vi "KM Lockin.vi"() -> ()   [LabVIEW 2015]
uses:
  MQM Data Transfer_KM.vi
  String Array Select.vi
  <vilib>/Utility/file.llb/Write To Spreadsheet File (string).vi
  Numeric Array Select.vi
  <vilib>/Utility/file.llb/Write To Spreadsheet File (DBL).vi
panel:
  in  "Tab Control":enum32{"Display Data", "Sweep Arming"}(tab)
  in  "Control":bool=TRUE
  in  "Stop":bool=TRUE
  out "XY Graph":cluster{dbl[], dbl[]}[](graph)
  in  "Display Elements":cluster{"X":bool, "Y":bool, "Name":u16}[](array[cluster]) {"Name" items=["Time (ms)", "Field (T)", "Temperature (K)", "", "HFLI_1.0 Freq (Hz)", "HFLI_1.0 R (V)", "HFLI_1.0 Theta (deg)", "HFLI_1.0 X (mV)", "HFLI_1.0 Y (mV)"]}
  in  "X-Axis":u16(ring) items=["Linear", "Reciprocal", "Log10"]
  in  "Filename":path=path "C:/Users/putkonen.CPFS/Dropbox.lvm"
  in  "Delay (ms)":dbl=2000.0
  out "Data Rate (ms)":u32
  in  "Finish":bool
  out "Measurement":bool
  in  "Y-Axis":u16(ring) items=["Linear", "Reciprocal", "Log10"]
  out "Saving":bool
  in  "Data Recording":bool=TRUE
  in  "DAQ time (ms)":u32=500
  out "Circles":cluster{dbl[], dbl[]}(graph)
  in  "X":u16(ring) items=["Linear", "Reciprocal", "Log10"]
  in  "Y":u16(ring) items=["Linear", "Reciprocal", "Log10"]
  out "Phase":cluster{dbl[], dbl[]}(graph)
  in  "Frequency":u16(ring) items=["Linear", "Reciprocal", "Log10"]
  in  "Theta":u16(ring) items=["Linear", "Reciprocal", "Log10"]
  out "# pts in freq sweep":i32
  out "Data Rate  (ms)":u32
  in  "DAQ time (ms)":u32=50
  in  "Fequency sweep datafile":path=path "C:/Users/putkonen.CPFS/Dropbox.lvm" caption="Filename"
  in  "Save current freq scan":bool
  in  "Start (Hz)":dbl=48.29
  in  "Stop (Hz)":dbl=48.57
  in  "# pts in scan":dbl=100.0
  in  "Bandwidth (Hz)":dbl=10.0
  in  "Use Sweep Control":bool
  in  "Sweep Parameter":u16(ring) items=["Temperature", "Field", "Position", "Measure when stable"]
  out "Global Stop":bool
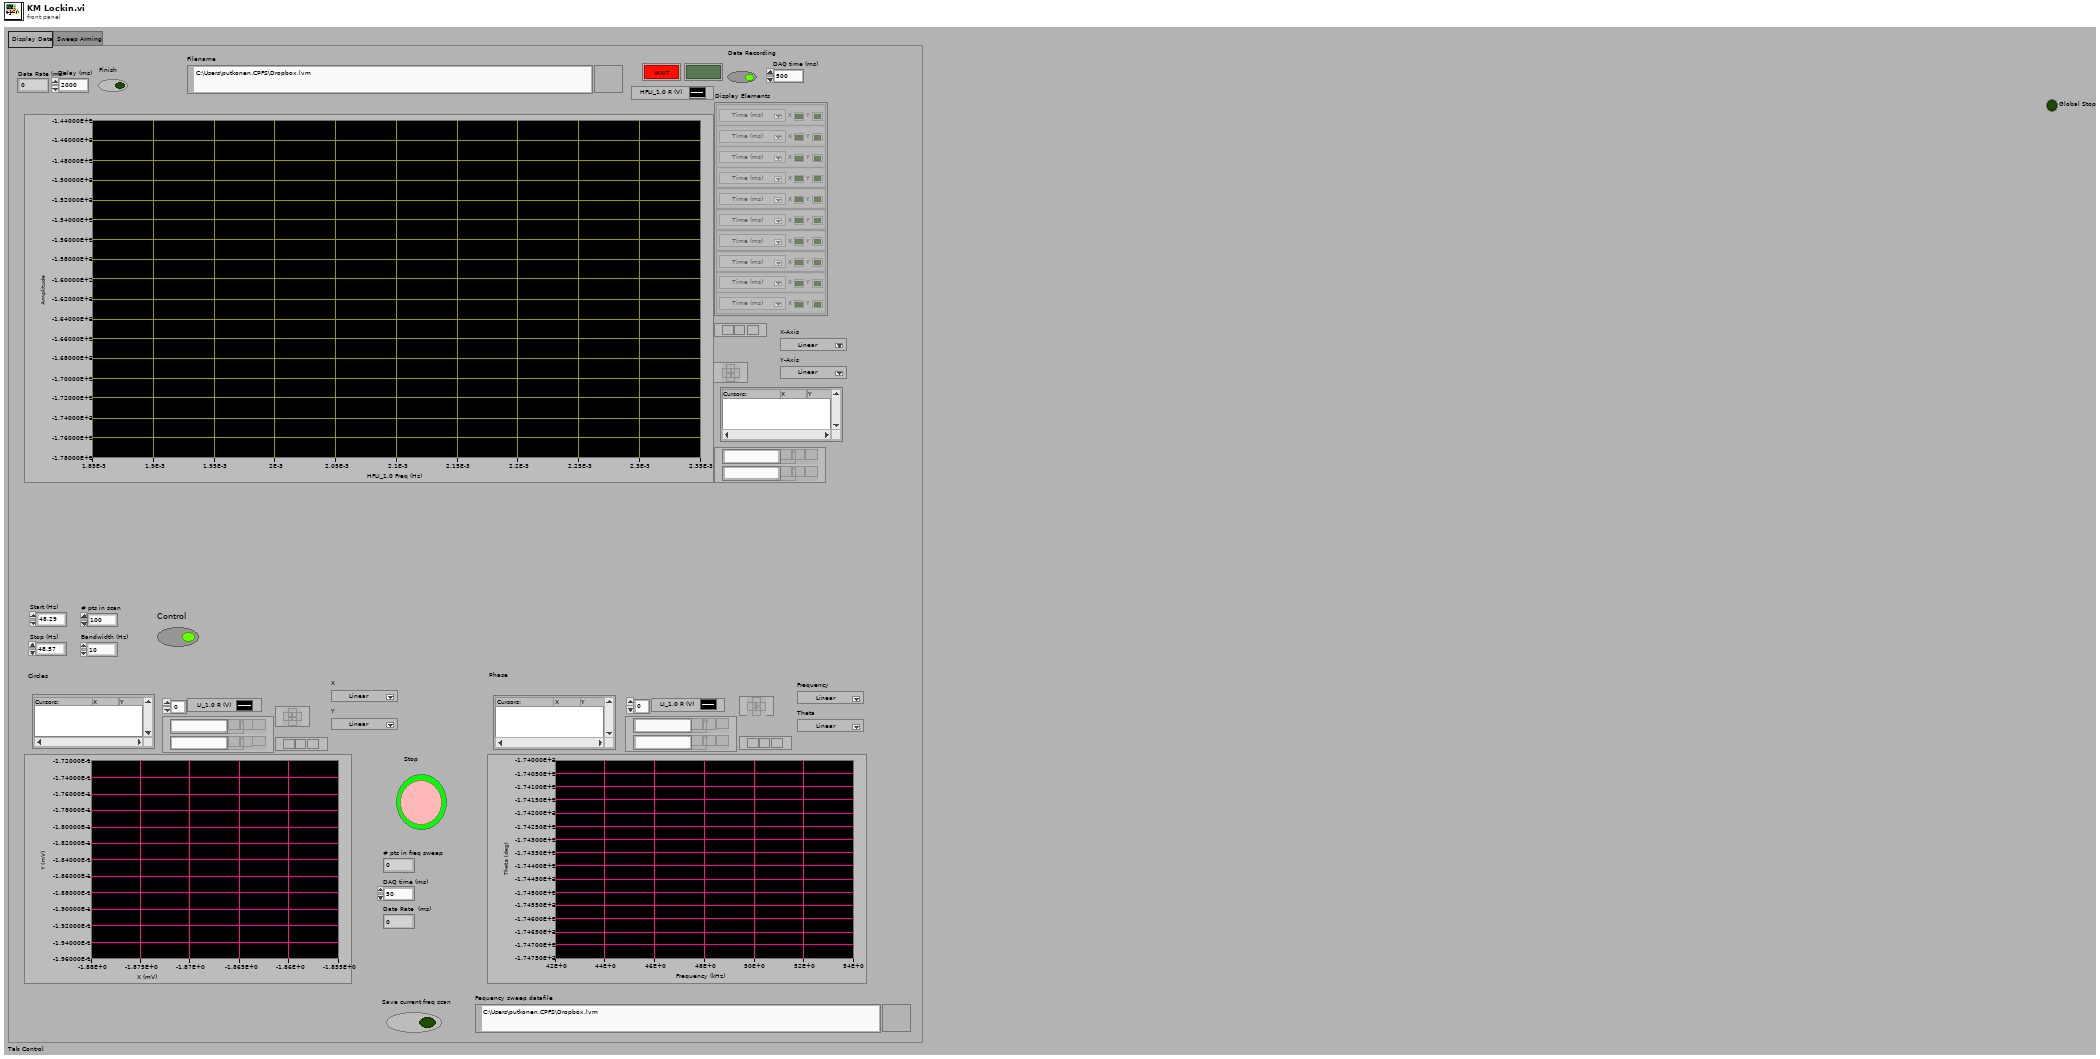
[diagram p1: front panel]
types:
  T1 = typedef "ZI_Frontpanel.ctl" = cluster{"Lockin 1 Demod 0":cluster{"R(V)":dbl, "Theta (deg)":dbl, "Timestamp (ms)":u32}, "Lockin 2 Demod 0":cluster{"R(V)":dbl, "Theta (deg)":dbl, "Timestamp (ms)":u32}, "Lockin 3 Demod 0":cluster{"R(V)":dbl, "Theta (deg)":dbl, "Timestamp (ms)":u32}, "Lockin 4 Demod 0":cluster{"R(V)":dbl, "Theta (deg)":dbl, "Timestamp (ms)":u32}, "Lockin 1 Demod 1":cluster{"R(V)":dbl, "Theta (deg)":dbl, "Timestamp (ms)":u32}, "Lockin 2 Demod 1":cluster{"R(V)":dbl, "Theta (deg)":dbl, "Timestamp (ms)":u32}, "Lockin 3 Demod 1":cluster{"R(V)":dbl, "Theta (deg)":dbl, "Timestamp (ms)":u32}, "Lockin 4 Demod 1":cluster{"R(V)":dbl, "Theta (deg)":dbl, "Timestamp (ms)":u32}, "Lockin 1 Demod 2":cluster{"R(V)":dbl, "Theta (deg)":dbl, "Timestamp (ms)":u32}, "Lockin 1 Demod 3":cluster{"R(V)":dbl, "Theta (deg)":dbl, "Timestamp (ms)":u32}, "LI1 active":bool, "LI2 active":bool, "LI3 active":bool, "LI4 active":bool}
  T2 = typedef "PPMS_Status.ctl" = cluster{"Field":cluster{"Field (T)":dbl, "Field stable":bool, "Timestamp (ms)":u32}, "Temperature":cluster{"Temperature (K)":dbl, "Temperature stable":bool, "Timestamp (ms)":u32}}
  T3 = typedef "Rotator_Status.ctl" = cluster{"Angle (deg)":dbl, "Stopped":bool, "Timestamp (ms)":u32}
  T4 = cluster{"Request new file":bool, "Sweep variable":u16, "Pause DAQ":bool}
  T5 = typedef "HF_FrontPanel.ctl" = cluster{"Lockin 1 Demod 0":cluster{"R(V)":dbl, "Theta (deg)":dbl, "Frequency (Hz)":dbl, "X (mV)":dbl, "Y (mV)":dbl}, "LI1 active":bool, "Timestamp (ms)":u32}
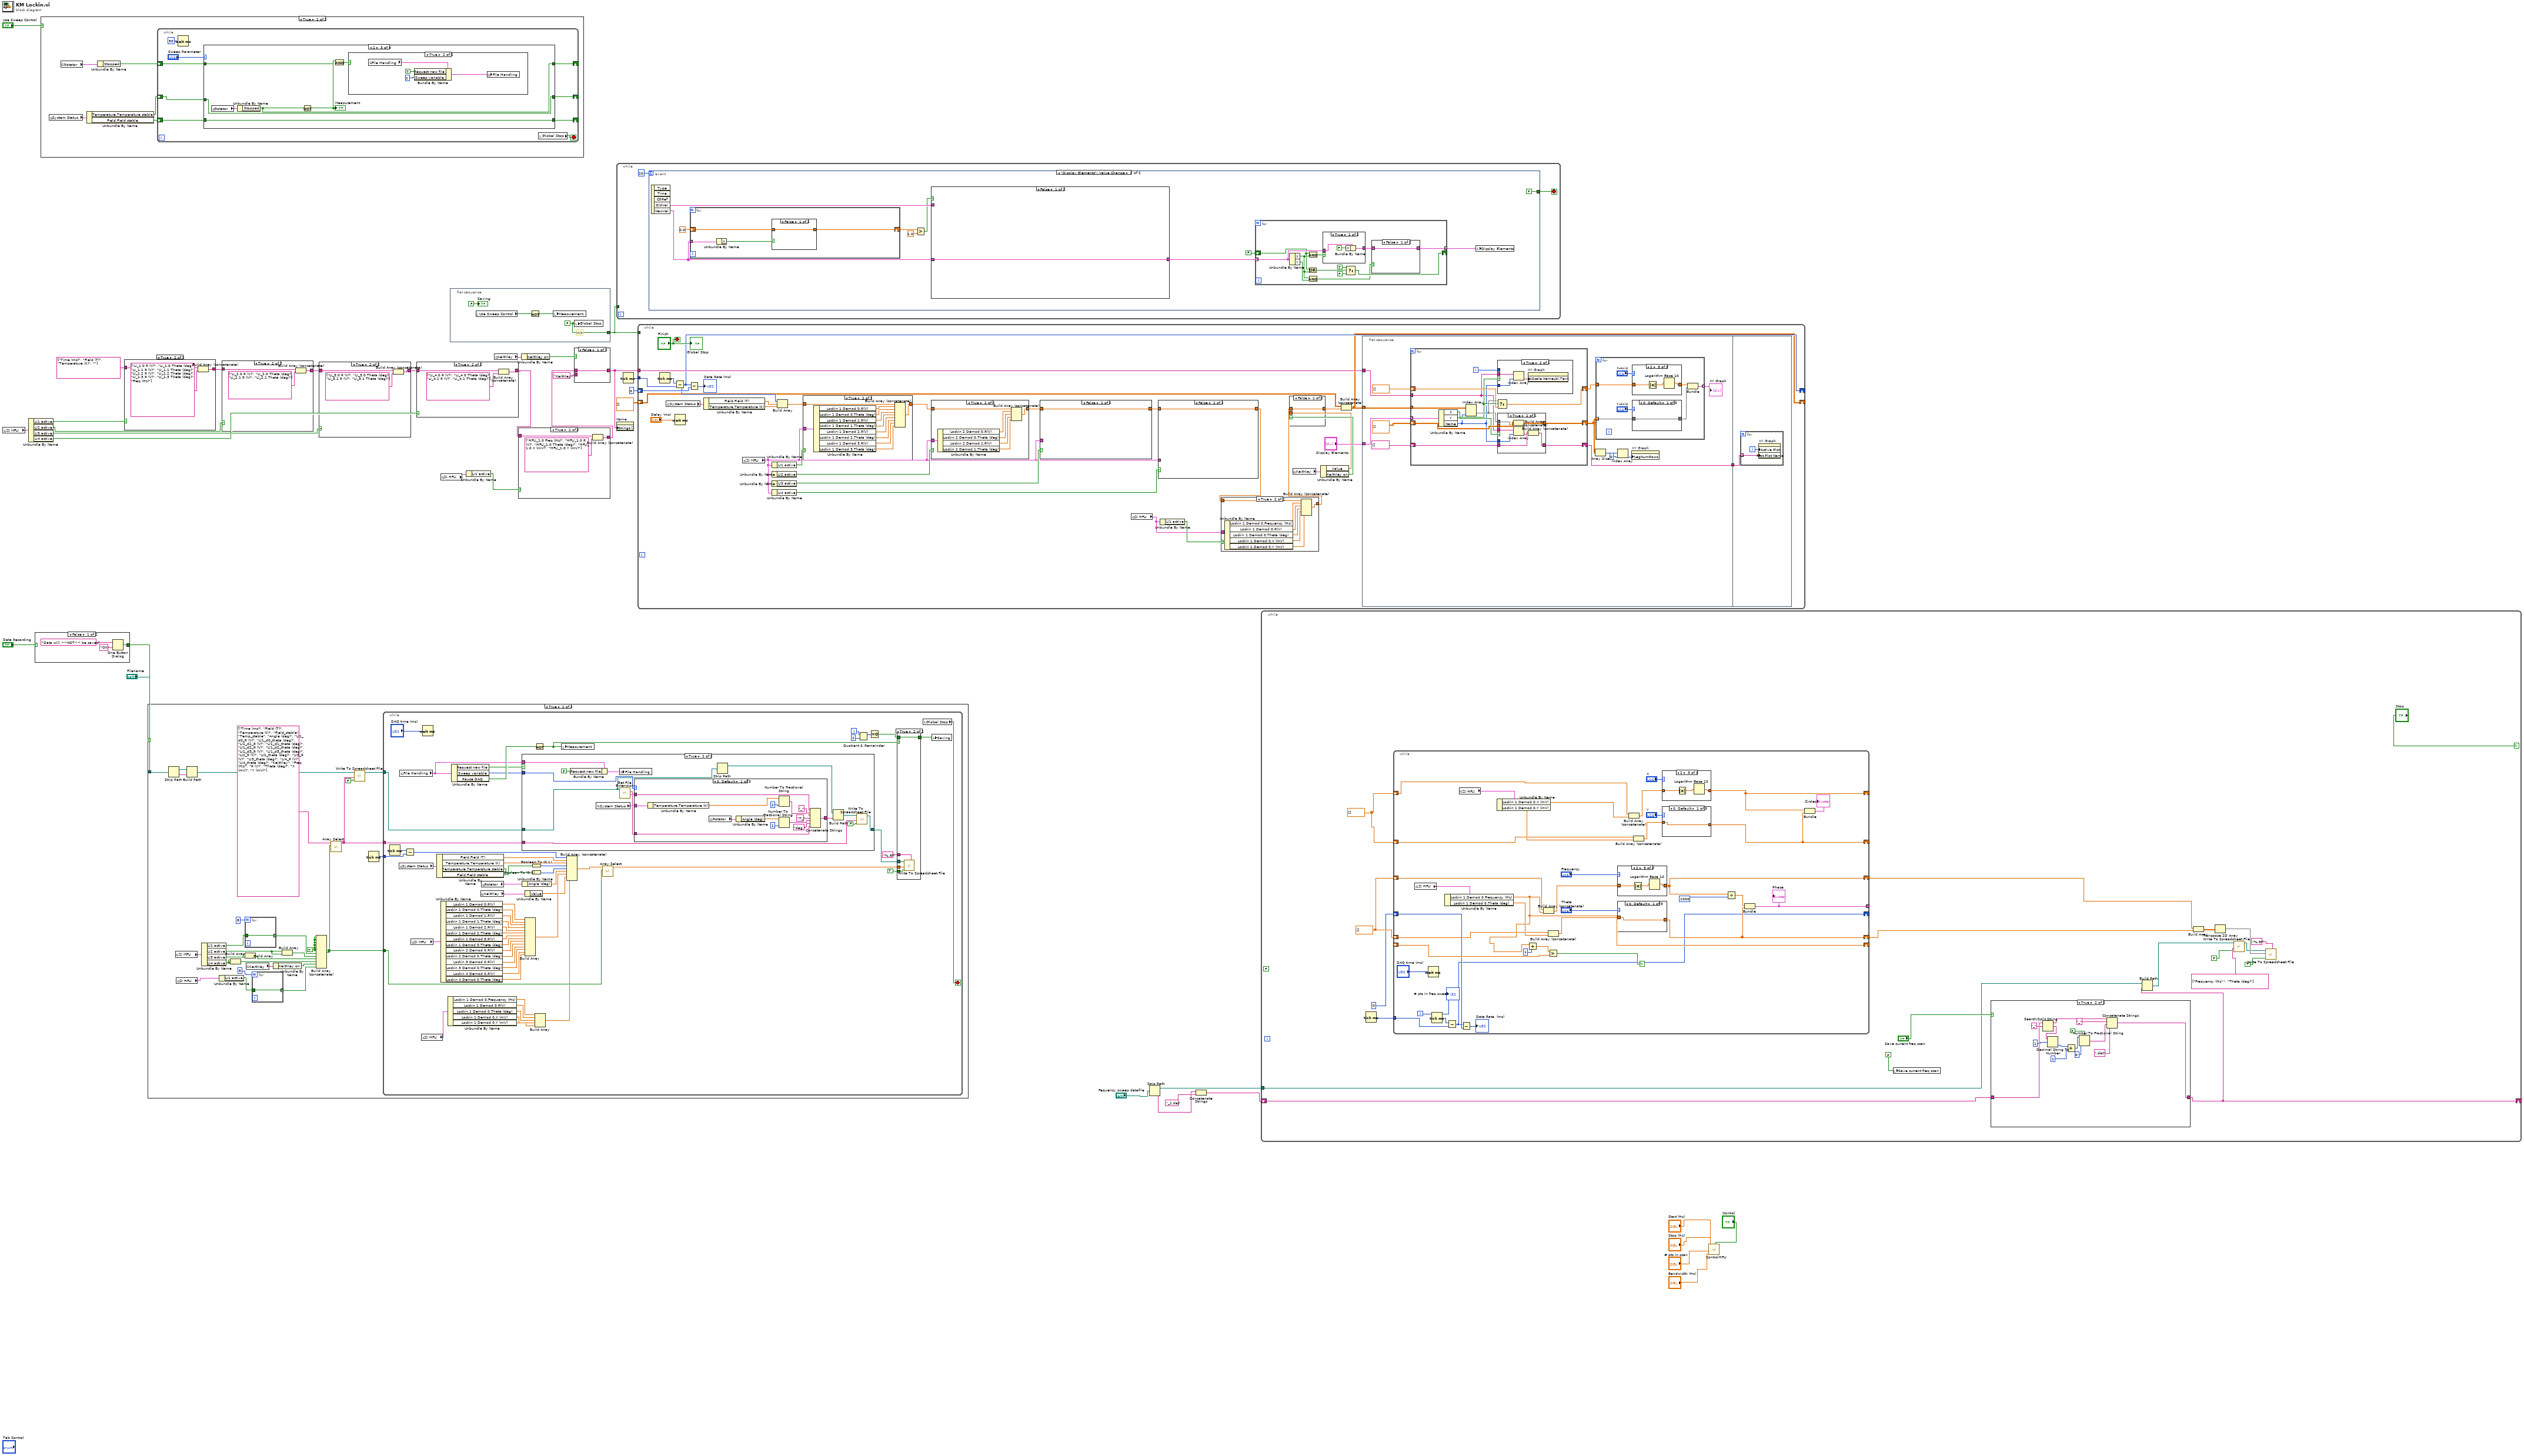
[diagram p0: block diagram]
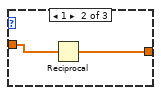
[diagram p3: hidden frame]
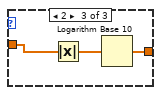
[diagram p4: hidden frame]
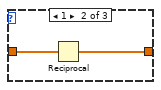
[diagram p6: hidden frame]
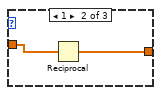
[diagram p7: hidden frame]
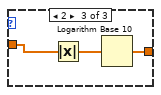
[diagram p8: hidden frame]
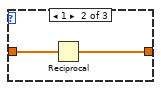
[diagram p10: hidden frame]
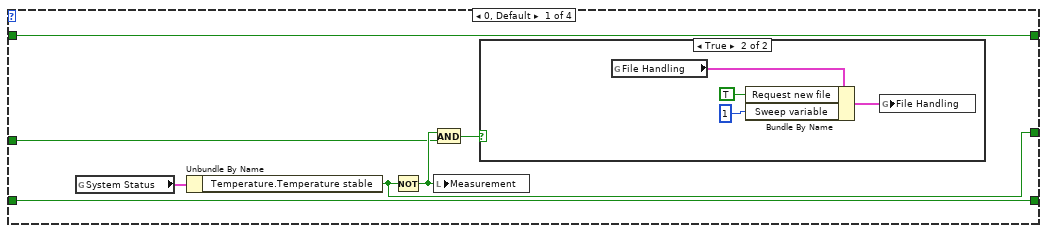
[diagram p13: hidden frame]
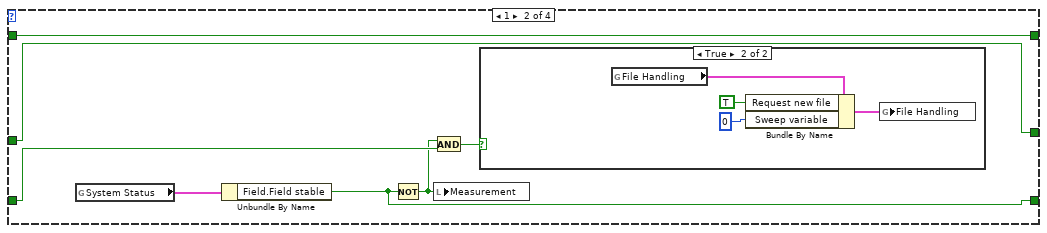
[diagram p15: hidden frame]
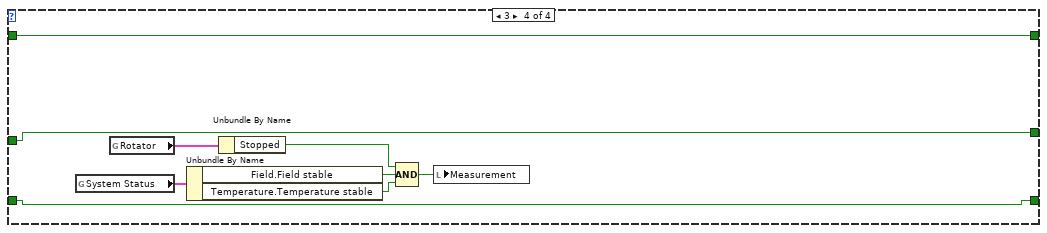
[diagram p18: hidden frame]
diagram:
  n1 = global read "MQM Data Transfer_KM.vi" "ZI MFLI"() -> (w33:T1)
  n2 = Unbundle By Name(w33) -> ("LI1 active"=w32:bool, "LI2 active"=w30:bool, "LI3 active"=w24:bool, "LI4 active"=w23:bool)
  n3 = case shown="False" "Data Recording" {
    selector: "Data Recording" -> [_ w39]
    tunnel: [w36 w39] -> w17
    frame False {
      n4 = One Button Dialog(message="Data will >>NOT<< be saved", button name ("OK")="OK") -> (true=w36:bool)
    }
    frame True {
    }
  }
  n5 = case shown="True" "Use Sweep Control" {
    frame False {
    }
    frame True {
      n6 = global read "MQM Data Transfer_KM.vi" "System Status"() -> (w42:T2)
      n7 = global read "MQM Data Transfer_KM.vi" "Rotator"() -> (w44:T3)
      n8 = Unbundle By Name(w42) -> ("Temperature.Temperature stable"=w41:bool, "Field.Field stable"=w40:bool)
      n9 = Unbundle By Name(w44) -> ("Stopped"=w43:bool)
      n10 = while {
        shift-right: [w51] -> _
        shift-left: w43 -> [w50]
        shift-right: [w48] -> _
        shift-left: w41 -> [w49]
        shift-right: [w47] -> _
        shift-left: w40 -> [w46]
        stop <- w45 stop-if-true
        n11 = Wait (ms)(milliseconds to wait=u32 50) -> ()  [unwired: 1 out]
        n12 = case shown="2" "Sweep Parameter" {
          tunnel: [w59 w69 w81 w89] -> w51
          tunnel: w50 -> [w59 w69 w79 w89]
          tunnel: w49 -> [w56 w70 w77 w88]
          tunnel: [w58 w70 w77 w88] -> w48
          tunnel: [w54 w66 w76 w87] -> w47
          tunnel: w46 -> [w54 w67 w76 w87]
          frame 0, Default {
            n13 = global read "MQM Data Transfer_KM.vi" "System Status"() -> (w60:T2)
            n14 = Unbundle By Name(w60) -> ("Temperature.Temperature stable"=w58:bool)
            n15 = Not(x=w58) -> (.not. x?=w57:bool)
            n16 = And(x=w57, y=w56) -> (x .and. y?=w55:bool)
            n17 = local write "Measurement"(w57) -> ()
            n18 = case shown="True" w55 {
              frame False {
              }
              frame True {
                n19 = global read "MQM Data Transfer_KM.vi" "File Handling"() -> (w64:T4)
                n20 = Bundle By Name(cluster=w64, "Request new file"=TRUE, "Sweep variable"=u16 1) -> (w63:T4)
                n21 = global write "MQM Data Transfer_KM.vi" "File Handling"(w63) -> ()
              }
            }
          }
          frame 1 {
            n22 = global read "MQM Data Transfer_KM.vi" "System Status"() -> (w71:T2)
            n23 = Unbundle By Name(w71) -> ("Field.Field stable"=w66:bool)
            n24 = Not(x=w66) -> (.not. x?=w65:bool)
            n25 = And(x=w65, y=w67) -> (x .and. y?=w68:bool)
            n26 = local write "Measurement"(w65) -> ()
            n27 = case shown="True" w68 {
              frame False {
              }
              frame True {
                n28 = global read "MQM Data Transfer_KM.vi" "File Handling"() -> (w75:T4)
                n29 = Bundle By Name(cluster=w75, "Request new file"=TRUE, "Sweep variable"=u16 0) -> (w74:T4)
                n30 = global write "MQM Data Transfer_KM.vi" "File Handling"(w74) -> ()
              }
            }
          }
          frame 2 {
            n31 = global read "MQM Data Transfer_KM.vi" "Rotator"() -> (w82:T3)
            n32 = Unbundle By Name(w82) -> ("Stopped"=w81:bool)
            n33 = Not(x=w81) -> (.not. x?=w80:bool)
            "Measurement" <- w80
            n34 = And(x=w80, y=w79) -> (x .and. y?=w78:bool)
            n35 = case shown="True" w78 {
              frame False {
              }
              frame True {
                n36 = global read "MQM Data Transfer_KM.vi" "File Handling"() -> (w86:T4)
                n37 = Bundle By Name(cluster=w86, "Request new file"=TRUE, "Sweep variable"=u16 2) -> (w85:T4)
                n38 = global write "MQM Data Transfer_KM.vi" "File Handling"(w85) -> ()
              }
            }
          }
          frame 3 {
            n39 = global read "MQM Data Transfer_KM.vi" "System Status"() -> (w93:T2)
            n40 = global read "MQM Data Transfer_KM.vi" "Rotator"() -> (w95:T3)
            n41 = Unbundle By Name(w93) -> ("Field.Field stable"=w92:bool, "Temperature.Temperature stable"=w91:bool)
            n42 = Unbundle By Name(w95) -> ("Stopped"=w94:bool)
            n43 = Compound Arithmetic op=AND(w94, w92, w91) -> (w90:bool)
            n44 = local write "Measurement"(w90) -> ()
          }
        }
        n45 = local read "Global Stop"() -> (w45:bool)
      }
    }
  }
  n46 = case shown="True" w32 {
    tunnel: string[] ["Time (ms)", "Field (T)", "Temperature (K)", ""] -> [w96 w99]
    tunnel: [w96 w97] -> w29
    frame False {
    }
    frame True {
      n47 = Build Array (concatenate)(w99, string[] ["LI_1.0 R (V)", "LI_1.0 Theta (deg)", "LI_1.1 R (V)", "LI_1.1 Theta (deg)", "LI_1.2 R (V)", "LI_1.2 Theta (deg)", "LI_1.3 R (V)", "LI_1.3 Theta (deg)", "Freq (Hz)"]) -> (w97:string[])
    }
  }
  n48 = case shown="True" w17 {
    tunnel: "Filename" -> [_ w126]
    frame False {
    }
    frame True {
      w118 = TRUE
      n49 = Strip Path(path=w126) -> (stripped path=w122:path, name=w120:string)
      n50 = global read "MQM Data Transfer_KM.vi" "ZI MFLI"() -> (w117:T1)
      n51 = global read "MQM Data Transfer_KM.vi" "ZI HFLI"() -> (w103:T5)
      n52 = Build Path(base path=w122, name or relative path=w120) -> (appended path=w123:path)
      n53 = Unbundle By Name(w117) -> ("LI1 active"=w116:bool, "LI2 active"=w113:bool, "LI3 active"=w112:bool, "LI4 active"=w111:bool)
      n54 = Unbundle By Name(w103) -> ("LI1 active"=w102:bool)
      n55 = Build Array(w111, w111) -> (w108:bool[])
      n56 = for {
        N: 8 -> [_]
        tunnel: w116 -> [w128]
        tunnel: [w128] -> w114 mode=indexing
      }
      n57 = Build Array(w112, w112) -> (w109:bool[])
      n58 = global read "MQM Data Transfer_KM.vi" "Keithley"() -> (w107:cluster{"Value":dbl, "Keithley on":bool})
      n59 = for {
        N: 5 -> [_]
        tunnel: w102 -> [w127]
        tunnel: [w127] -> w100 mode=indexing
      }
      n60 = Unbundle By Name(w107) -> ("Keithley on"=w106:bool)
      n61 = Build Array(w113, w113) -> (w110:bool[])
      n62 = Build Array (concatenate)(w118, w118, w118, w118, w118, w118, w114, w110, w109, w108, w106, w100) -> (w105:bool[])
      n63 = call-poly "Array Select.vi"("Selector array"=w105, "Full array"=string[] ["Time (ms)", "Field (T)", "Temperature (K)", "Field_stable", "Temp_stable", "Angle (deg)", "LI1_d0_R (V)", "LI1_d0_theta (deg)", "LI1_d1_R (V)", "LI1_d1_theta (deg)", "LI1_d2_R (V)", "LI1_d2_theta (deg)", "LI1_d3_R (V)", "LI1_d3_theta (deg)", "LI2_R (V)", "LI2_theta (deg)", "LI3_R (V)", "LI3_theta (deg)", "LI4_R (V)", "LI4_theta (deg)", "Keithley", "Freq (Hz)", "R (V)", "Theta (deg)", "X (mV)", "Y (mV)"]) -> ("Array"=w104:string[])  [unwired: 9 in]
      n64 = call-poly <vilib>:"Write To Spreadsheet File.vi"("append to file? (new file:F)"=FALSE, "1D data"=w104, "file path (dialog if empty)"=w123) -> ("new file path (Not A Path if cancelled)"=w121:path)  [unwired: 5 in]
      n65 = Tick Count (ms)() -> (millisecond timer value=w125:u32)
      n66 = while {
        tunnel: w125 -> [w185]
        tunnel: w121 -> [w143]
        tunnel: w105 -> [w152]
        tunnel: w104 -> [w140]
        i -> [w151]
        stop <- w177 stop-if-true
        n67 = Tick Count (ms)() -> (millisecond timer value=w183:u32)
        n68 = global read "MQM Data Transfer_KM.vi" "System Status"() -> (w184:T2)
        n69 = global read "MQM Data Transfer_KM.vi" "File Handling"() -> (w139:T4)
        n70 = Subtract(x=w183, y=w185) -> (x-y=w182:u32)
        n71 = global read "MQM Data Transfer_KM.vi" "ZI MFLI"() -> (w173:T1)
        n72 = global read "MQM Data Transfer_KM.vi" "ZI HFLI"() -> (w136:T5)
        n73 = Wait (ms)(milliseconds to wait="DAQ time (ms)") -> ()  [unwired: 1 out]
        n74 = Unbundle By Name(w184) -> ("Field.Field (T)"=w181:dbl, "Temperature.Temperature (K)"=w180:dbl, "Temperature.Temperature stable"=w161:bool, "Field.Field stable"=w163:bool)
        n75 = Unbundle By Name(w173) -> ("Lockin 1 Demod 0.R(V)"=w172:dbl, "Lockin 1 Demod 0.Theta (deg)"=w171:dbl, "Lockin 1 Demod 1.R(V)"=w170:dbl, "Lockin 1 Demod 1.Theta (deg)"=w169:dbl, "Lockin 1 Demod 2.R(V)"=w168:dbl, "Lockin 1 Demod 2.Theta (deg)"=w167:dbl, "Lockin 1 Demod 3.R(V)"=w166:dbl, "Lockin 1 Demod 3.Theta (deg)"=w165:dbl, "Lockin 2 Demod 0.R(V)"=w164:dbl, "Lockin 2 Demod 0.Theta (deg)"=w157:dbl, "Lockin 3 Demod 0.R(V)"=w156:dbl, "Lockin 3 Demod 0.Theta (deg)"=w155:dbl, "Lockin 4 Demod 0.R(V)"=w154:dbl, "Lockin 4 Demod 0.Theta (deg)"=w153:dbl)
        n76 = Unbundle By Name(w136) -> ("Lockin 1 Demod 0.Frequency (Hz)"=w135:dbl, "Lockin 1 Demod 0.R(V)"=w134:dbl, "Lockin 1 Demod 0.Theta (deg)"=w133:dbl, "Lockin 1 Demod 0.X (mV)"=w132:dbl, "Lockin 1 Demod 0.Y (mV)"=w131:dbl)
        n77 = Unbundle By Name(w139) -> ("Request new file"=w144:bool, "Sweep variable"=w141:u16, "Pause DAQ"=w148:bool)
        n78 = global read "MQM Data Transfer_KM.vi" "Keithley"() -> (w174:cluster{"Value":dbl, "Keithley on":bool})
        n79 = global read "MQM Data Transfer_KM.vi" "Rotator"() -> (w175:T3)
        n80 = case shown="True" w144 {
          tunnel: w143 -> [w186 w197]
          tunnel: [w186 w190] -> w142
          tunnel: w141 -> [_ w199]
          tunnel: w140 -> [_ w192]
          tunnel: w139 -> [_ w189]
          frame False {
          }
          frame True {
            n81 = Bundle By Name(cluster=w189, "Request new file"=FALSE) -> (w187:T4)
            n82 = global read "MQM Data Transfer_KM.vi" "System Status"() -> (w198:T2)
            n83 = global write "MQM Data Transfer_KM.vi" "File Handling"(w187) -> ()
            n84 = call <vilib>:"Get File Extension.vi"("file"=w197) -> ("filename without extension"=w196:string, "lowercase file extension"=w195:string)  [unwired: 6 in, 3 out]
            n85 = case shown="0, Default" w199 {
              tunnel: w198 -> [w214 w223 w234]
              tunnel: w196 -> [w211 w224 w236]
              tunnel: w195 -> [w201 w215 w229]
              tunnel: [w207 w221 w235] -> w194
              frame 0, Default {
                n86 = Unbundle By Name(w214) -> ("Temperature.Temperature (K)"=w213:dbl)
                n87 = global read "MQM Data Transfer_KM.vi" "Rotator"() -> (w206:T3)
                n88 = Unbundle By Name(w206) -> ("Angle (deg)"=w204:dbl)
                n89 = Number To Fractional String(number=w213, precision (6)=i16 2) -> (F-format string=w209:string)  [unwired: 2 in]
                n90 = Number To Fractional String(number=w204, precision (6)=i16 1) -> (F-format string=w203:string)  [unwired: 2 in]
                n91 = Concatenate Strings(w211, "_", w209, "T_", w203, "deg." ("string"), w201) -> (w207:string)
              }
              frame 1 {
                n92 = Unbundle By Name(w223) -> ("Field.Field (T)"=w222:dbl)
                n93 = global read "MQM Data Transfer_KM.vi" "Rotator"() -> (w220:T3)
                n94 = Unbundle By Name(w220) -> ("Angle (deg)"=w218:dbl)
                n95 = Number To Fractional String(number=w222, precision (6)=i16 2) -> (F-format string=w226:string)  [unwired: 2 in]
                n96 = Number To Fractional String(number=w218, precision (6)=i16 1) -> (F-format string=w217:string)  [unwired: 2 in]
                n97 = Concatenate Strings(w224, "_", w226, "T_", w217, "deg." ("string"), w215) -> (w221:string)
              }
              frame 2 {
                n98 = Unbundle By Name(w234) -> ("Field.Field (T)"=w241:dbl, "Temperature.Temperature (K)"=w232:dbl)
                n99 = Number To Fractional String(number=w241, precision (6)=i16 2) -> (F-format string=w238:string)  [unwired: 2 in]
                n100 = Number To Fractional String(number=w232, precision (6)=i16 2) -> (F-format string=w231:string)  [unwired: 2 in]
                n101 = Concatenate Strings(w236, "_", w238, "T_", w231, "K." ("string"), w229) -> (w235:string)
              }
            }
            n102 = Strip Path(path=w197) -> (stripped path=w200:path)  [unwired: 1 out]
            n103 = Build Path(base path=w200, name or relative path=w194) -> (appended path=w191:path)
            n104 = call-poly <vilib>:"Write To Spreadsheet File.vi"("append to file? (new file:F)"=FALSE, "1D data"=w192, "file path (dialog if empty)"=w191) -> ("new file path (Not A Path if cancelled)"=w190:path)  [unwired: 5 in]
          }
        }
        n105 = Unbundle By Name(w175) -> ("Angle (deg)"=w159:dbl)
        n106 = Build Array(w172, w171, w170, w169, w168, w167, w166, w165, w164, w157, w156, w155, w154, w153) -> (w158:dbl[])
        n107 = Unbundle By Name(w174) -> ("Value"=w137:dbl)
        n108 = Boolean To (0,1)(Boolean=w163) -> (0, 1=w162:i16)
        n109 = Boolean To (0,1)(Boolean=w161) -> (0, 1=w160:i16)
        n110 = Not(x=w148) -> (.not. x?=w147:bool)
        n111 = Build Array(w135, w134, w133, w132, w131) -> (w130:dbl[])
        n112 = local write "Measurement"(w147) -> ()
        n113 = Build Array (concatenate)(w182, w181, w180, w162, w160, w159, w158, w137, w130) -> (w138:dbl[])
        n114 = call-poly "Array Select.vi"("Selector array"=w152, "Full array"=w138) -> ("Array"=w129:dbl[])  [unwired: 9 in]
        n115 = Quotient & Remainder(x=w151, y=2) -> (x-y*floor(x/y)=w149:i32)  [unwired: 1 out]
        n116 = Equal To 0?(x=w149) -> (x = 0?=w146:bool)
        n117 = case shown="True" w147 {
          tunnel: TRUE ("append to file? (new file:F)") -> [_ w247]
          tunnel: "%.8f" ("format (%.3f)") -> [_ w246]
          tunnel: w129 -> [_ w245]
          tunnel: w146 -> [_ w244]
          tunnel: [FALSE w244] -> w145
          tunnel: w142 -> [_ w243]
          frame False {
          }
          frame True {
            n118 = call-poly <vilib>:"Write To Spreadsheet File.vi"("format (%.3f)"=w246, "append to file? (new file:F)"=w247, "1D data"=w245, "file path (dialog if empty)"=w243) -> ()  [unwired: 4 in, 1 out]
          }
        }
        n119 = local read "Global Stop"() -> (w177:bool)
        n120 = local write "Saving"(w145) -> ()
      }
    }
  }
  n121 = case shown="True" w30 {
    tunnel: w29 -> [w248 w251]
    tunnel: [w248 w249] -> w28
    frame False {
    }
    frame True {
      n122 = Build Array (concatenate)(w251, string[] ["LI_2.0 R (V)", "LI_2.0 Theta (deg)", "LI_2.1 R (V)", "LI_2.1 Theta (deg)"]) -> (w249:string[])
    }
  }
  n123 = case shown="True" w24 {
    tunnel: w28 -> [w252 w255]
    tunnel: [w252 w253] -> w27
    frame False {
    }
    frame True {
      n124 = Build Array (concatenate)(w255, string[] ["LI_3.0 R (V)", "LI_3.0 Theta (deg)", "LI_3.1 R (V)", "LI_3.1 Theta (deg)"]) -> (w253:string[])
    }
  }
  n125 = case shown="True" w23 {
    tunnel: w27 -> [w256 w259]
    tunnel: [w256 w258] -> w12
    frame False {
    }
    frame True {
      n126 = Build Array (concatenate)(w259, string[] ["LI_4.0 R (V)", "LI_4.0 Theta (deg)", "LI_4.1 R (V)", "LI_4.1 Theta (deg)"]) -> (w258:string[])
    }
  }
  n127 = global read "MQM Data Transfer_KM.vi" "ZI HFLI"() -> (w14:T5)
  n128 = flat-sequence {
    tunnel: [w263] -> w25
    frame #0 {
      w263 = FALSE ("Global Stop")
      # "Init"
      n129 = local read "Use Sweep Control"() -> (w261:bool)
      n130 = Not(x=w261) -> (.not. x?=w260:bool)
      n131 = local write "Measurement"(w260) -> ()
      n132 = local write "Global Stop"(w263) -> ()
      "Saving" <- FALSE ("Saving")
    }
  }
  n133 = Unbundle By Name(w14) -> ("LI1 active"=w13:bool)
  n134 = global read "MQM Data Transfer_KM.vi" "Keithley"() -> (w20:cluster{"Value":dbl, "Keithley on":bool})
  n135 = case shown="True" w13 {
    tunnel: w12 -> [w264 w267]
    tunnel: [w264 w265] -> w11
    frame False {
    }
    frame True {
      n136 = Build Array (concatenate)(w267, string[] ["HFLI_1.0 Freq (Hz)", "HFLI_1.0 R (V)", "HFLI_1.0 Theta (deg)", "HFLI_1.0 X (mV)", "HFLI_1.0 Y (mV)"]) -> (w265:string[])
    }
  }
  n137 = Unbundle By Name(w20) -> ("Keithley on"=w19:bool)
  n138 = case shown="False" w19 {
    tunnel: w11 -> [w268 w271]
    tunnel: "Keithley" -> [_ w270]
    tunnel: [w268 w269] -> w21
    frame False {
    }
    frame True {
      n139 = Build Array (concatenate)(w271, w270) -> (w269:string[])
    }
  }
  n140 = while {
    tunnel: w25 -> [_]
    stop <- w272 stop-if-true
    n141 = event shown="[1] \"Display Elements\": Value Change" {
      selector: _ -> [_ _]
      dyn-events: _ -> [_ _]
      timeout: 20 -> [_ _]
      tunnel: [w274 FALSE] -> w272
      event Timeout {
        n142 = event-data() -> ()  [unwired: 1 in, 2 out]
        n143 = local read "Global Stop"() -> (w275:bool)
        n144 = case shown="False" w275 {
          tunnel: [FALSE TRUE] -> w274
          frame False {
          }
          frame True {
          }
        }
      }
      event "Display Elements": Value Change {
        n145 = event-data() -> ("OldVal"=w285:cluster{"X":bool, "Y":bool, "Name":u16}[], "NewVal"=w283:cluster{"X":bool, "Y":bool, "Name":u16}[])  [unwired: 1 in, 3 out]
        n146 = for {
          tunnel: w283 -> [w308] mode=indexing
          shift-right: [w306] -> w281
          shift-left: 0.0 -> [w305]
          n147 = Unbundle By Name(w308) -> ("X"=w307:bool)
          n148 = case shown="False" w307 {
            tunnel: [w309 w311] -> w306
            tunnel: w305 -> [w309 w310]
            frame False {
            }
            frame True {
              n149 = Increment(x=w310) -> (x+1=w311:dbl)
            }
          }
        }
        n150 = Greater?(x=w281, y=1.0) -> (0:w279:bool)
        n151 = case shown="False" w279 {
          tunnel: w285 -> [_ w291]
          tunnel: [w288 w290] -> w284
          tunnel: w283 -> [w288 w289]
          frame False {
          }
          frame True {
            n152 = for {
              tunnel: w289 -> [w294] mode=indexing
              tunnel: w291 -> [w298] mode=indexing
              tunnel: [w293] -> w290 mode=indexing
              n153 = Unbundle By Name(w298) -> ("X"=w297:bool)
              n154 = Unbundle By Name(w294) -> ("X"=w296:bool)
              n155 = Not(x=w297) -> (.not. x?=w295:bool)
              n156 = And(x=w295, y=w296) -> (x .and. y?=w292:bool)
              n157 = case shown="True" w292 {
                tunnel: [w299 w303] -> w293
                tunnel: w294 -> [w301 w302]
                frame False {
                  n158 = Bundle By Name(cluster=w301, "X"=FALSE) -> (w299:cluster{"X":bool, "Y":bool, "Name":u16})
                }
                frame True {
                  n159 = Bundle By Name(cluster=w302, "X"=TRUE) -> (w303:cluster{"X":bool, "Y":bool, "Name":u16})
                }
              }
            }
          }
        }
        n160 = for {
          tunnel: w284 -> [w322] mode=indexing
          shift-right: [w318] -> _
          shift-left: FALSE ("X") -> [w321]
          tunnel: [w312] -> w286 mode=indexing
          n161 = Unbundle By Name(w322) -> ("X"=w316:bool, "Y"=w315:bool)
          n162 = Or(x=w321, y=w316) -> (x .or. y?=w320:bool)
          n163 = And(x=w321, y=w316) -> (x .and. y?=w323:bool)
          n164 = And(x=w316, y=w315) -> (x .and. y?=w314:bool)
          n165 = case shown="True" w323 {
            tunnel: w322 -> [w328 w331]
            tunnel: [w328 w329] -> w313
            frame False {
            }
            frame True {
              n166 = Bundle By Name(cluster=w331, "X"=FALSE) -> (w329:cluster{"X":bool, "Y":bool, "Name":u16})
            }
          }
          n167 = Select(t=TRUE, s=w320, f=FALSE) -> (s? t:f=w318:bool)
          n168 = case shown="False" w314 {
            tunnel: w313 -> [w324 w327]
            tunnel: [w324 w326] -> w312
            frame False {
            }
            frame True {
              n169 = Bundle By Name(cluster=w327, "Y"=FALSE) -> (w326:cluster{"X":bool, "Y":bool, "Name":u16})
            }
          }
        }
        n170 = local write "Display Elements"(w286) -> ()
      }
    }
  }
  n171 = property on="Name" class="Ring (strict)"("Strings []"=w21) -> ()  [unwired: 2 in, 2 out]
  n172 = Tick Count (ms)() -> (millisecond timer value=w35:u32)
  n173 = while {
    tunnel: w35 -> [w362]
    shift-right: [w353] -> _
    shift-left: 0 -> [w361]
    tunnel: w21 -> [w355]
    shift-right: [w340] -> _
    shift-left: dbl[][] [] -> [w341]
    tunnel: w25 -> [_]
    stop <- "Finish" stop-if-true
    n174 = Tick Count (ms)() -> (millisecond timer value=w363:u32)
    n175 = global read "MQM Data Transfer_KM.vi" "System Status"() -> (w344:T2)
    n176 = Subtract(x=w363, y=w362) -> (x-y=w353:u32)
    n177 = Wait (ms)(milliseconds to wait="Delay (ms)") -> ()  [unwired: 1 out]
    n178 = Subtract(x=w353, y=w361) -> (x-y=→"Data Rate (ms)":u32)
    n179 = Unbundle By Name(w344) -> ("Field.Field (T)"=w343:dbl, "Temperature.Temperature (K)"=w342:dbl)
    n180 = global read "MQM Data Transfer_KM.vi" "ZI MFLI"() -> (w346:T1)
    n181 = Unbundle By Name(w346) -> ("LI1 active"=w354:bool)
    n182 = Unbundle By Name(w346) -> ("LI2 active"=w351:bool)
    n183 = Unbundle By Name(w346) -> ("LI3 active"=w349:bool)
    n184 = Unbundle By Name(w346) -> ("LI4 active"=w347:bool)
    n185 = Build Array(w353, w343, w342) -> (w352:dbl[])
    n186 = case shown="True" w354 {
      tunnel: w346 -> [_ w412]
      tunnel: w352 -> [w401 w411]
      tunnel: [w401 w402] -> w350
      frame False {
      }
      frame True {
        n187 = Unbundle By Name(w412) -> ("Lockin 1 Demod 0.R(V)"=w410:dbl, "Lockin 1 Demod 0.Theta (deg)"=w409:dbl, "Lockin 1 Demod 1.R(V)"=w408:dbl, "Lockin 1 Demod 1.Theta (deg)"=w407:dbl, "Lockin 1 Demod 2.R(V)"=w406:dbl, "Lockin 1 Demod 2.Theta (deg)"=w405:dbl, "Lockin 1 Demod 3.R(V)"=w404:dbl, "Lockin 1 Demod 3.Theta (deg)"=w403:dbl)
        n188 = Build Array (concatenate)(w411, w410, w409, w408, w407, w406, w405, w404, w403) -> (w402:dbl[])
      }
    }
    n189 = case shown="True" w351 {
      tunnel: w346 -> [_ w400]
      tunnel: w350 -> [w393 w395]
      tunnel: [w393 w394] -> w348
      frame False {
      }
      frame True {
        n190 = Unbundle By Name(w400) -> ("Lockin 2 Demod 0.R(V)"=w399:dbl, "Lockin 2 Demod 0.Theta (deg)"=w398:dbl, "Lockin 2 Demod 1.R(V)"=w397:dbl, "Lockin 2 Demod 1.Theta (deg)"=w396:dbl)
        n191 = Build Array (concatenate)(w395, w399, w398, w397, w396) -> (w394:dbl[])
      }
    }
    n192 = case shown="False" w349 {
      tunnel: w346 -> [_ w392]
      tunnel: w348 -> [w385 w387]
      tunnel: [w385 w386] -> w345
      frame False {
      }
      frame True {
        n193 = Unbundle By Name(w392) -> ("Lockin 3 Demod 0.R(V)"=w391:dbl, "Lockin 3 Demod 0.Theta (deg)"=w390:dbl, "Lockin 3 Demod 1.R(V)"=w389:dbl, "Lockin 3 Demod 1.Theta (deg)"=w388:dbl)
        n194 = Build Array (concatenate)(w387, w391, w390, w389, w388) -> (w386:dbl[])
      }
    }
    n195 = global read "MQM Data Transfer_KM.vi" "ZI HFLI"() -> (w334:T5)
    n196 = case shown="False" w347 {
      tunnel: w346 -> [_ w384]
      tunnel: w345 -> [w377 w379]
      tunnel: [w377 w378] -> w332
      frame False {
      }
      frame True {
        n197 = Unbundle By Name(w384) -> ("Lockin 4 Demod 0.R(V)"=w383:dbl, "Lockin 4 Demod 0.Theta (deg)"=w382:dbl, "Lockin 4 Demod 1.R(V)"=w381:dbl, "Lockin 4 Demod 1.Theta (deg)"=w380:dbl)
        n198 = Build Array (concatenate)(w379, w383, w382, w381, w380) -> (w378:dbl[])
      }
    }
    n199 = Unbundle By Name(w334) -> ("LI1 active"=w335:bool)
    n200 = case shown="True" w335 {
      tunnel: w334 -> [_ w372]
      tunnel: w332 -> [w364 w365]
      tunnel: [w364 w367] -> w333
      frame False {
      }
      frame True {
        n201 = Unbundle By Name(w372) -> ("Lockin 1 Demod 0.Frequency (Hz)"=w371:dbl, "Lockin 1 Demod 0.R(V)"=w370:dbl, "Lockin 1 Demod 0.Theta (deg)"=w369:dbl, "Lockin 1 Demod 0.X (mV)"=w368:dbl, "Lockin 1 Demod 0.Y (mV)"=w366:dbl)
        n202 = Build Array (concatenate)(w365, w371, w370, w369, w368, w366) -> (w367:dbl[])
      }
    }
    n203 = global read "MQM Data Transfer_KM.vi" "Keithley"() -> (w339:cluster{"Value":dbl, "Keithley on":bool})
    n204 = Unbundle By Name(w339) -> ("Value"=w338:dbl, "Keithley on"=w336:bool)
    n205 = case shown="False" w336 {
      tunnel: w333 -> [w373 w376]
      tunnel: w338 -> [_ w375]
      tunnel: [w373 w374] -> w337
      frame False {
      }
      frame True {
        n206 = Build Array (concatenate)(w376, w375) -> (w374:dbl[])
      }
    }
    n207 = Build Array (concatenate)(w341, w337) -> (w340:dbl[][])
    n208 = flat-sequence {
      tunnel: "Display Elements" -> [w415]
      tunnel: [w419] -> w359
      tunnel: w355 -> [w413]
      tunnel: w340 -> [w414]
      tunnel: w359 -> [w472]
      frame #0 {
        n209 = for {
          tunnel: w415 -> [w452] mode=indexing
          shift-right: [w458] -> w425
          shift-left: dbl[] [] -> [w457]
          shift-right: [w446] -> w423
          shift-left: dbl[][] [] -> [w454]
          shift-right: [w450] -> w419
          shift-left: string[] [] -> [w449]
          tunnel: w413 -> [w445]
          tunnel: w414 -> [w447]
          i -> [w448]
          n210 = Unbundle By Name(w452) -> ("X"=w453:bool, "Y"=w456:bool, "Name"=w451:u16)
          n211 = Index Array(array=w447, index (col)=w451) -> (element=w455:dbl[])  [unwired: 1 in]
          n212 = Select(t=w455, s=w453, f=w457) -> (s? t:f=w458:dbl[])
          n213 = case shown="True" w453 {
            tunnel: w451 -> [_ w461]
            tunnel: w448 -> [_ _]
            tunnel: w445 -> [_ w459]
            frame False {
            }
            frame True {
              n214 = Index Array(array=w459, index=w461) -> (element=w460:string)
              n215 = property on="XY Graph" class="XYGraph (strict)"("XScale.NameLbl.Text"=w460) -> ()  [unwired: 2 in, 2 out]
            }
          }
          n216 = case shown="True" w456 {
            tunnel: w455 -> [_ w464]
            tunnel: w454 -> [w462 w471]
            tunnel: [w462 w470] -> w446
            tunnel: w451 -> [_ w469]
            tunnel: [w463 w467] -> w450
            tunnel: w449 -> [w463 w466]
            tunnel: w445 -> [_ w465]
            frame False {
            }
            frame True {
              n217 = Build Array (concatenate)(w471, w464) -> (w470:dbl[][])
              n218 = Index Array(array=w465, index=w469) -> (element=w468:string)
              n219 = Build Array (concatenate)(w466, w468) -> (w467:string[])
            }
          }
        }
        n220 = Array Size(array=w423) -> (size(s)=w422:i32[])
        n221 = for {
          tunnel: w423 -> [w429] mode=indexing
          tunnel: w425 -> [w431]
          tunnel: [w432] -> w424 mode=indexing
          n222 = case shown="2" "X-Axis" {
            tunnel: w431 -> [w439 w441 w444]
            tunnel: [w439 w440 w443] -> w430
            frame 0, Default {
            }
            frame 1 {
              n223 = Reciprocal(x=w441) -> (1/x=w440:dbl[])
            }
            frame 2 {
              n224 = Absolute Value(x=w444) -> (abs(x)=w442:dbl[])
              n225 = Logarithm Base 10(1:w442) -> (0:w443:dbl[])
            }
          }
          n226 = case shown="0, Default" "Y-Axis" {
            tunnel: w429 -> [w433 w435 w438]
            tunnel: [w433 w434 w437] -> w426
            frame 0, Default {
            }
            frame 1 {
              n227 = Reciprocal(x=w435) -> (1/x=w434:dbl[])
            }
            frame 2 {
              n228 = Absolute Value(x=w438) -> (abs(x)=w436:dbl[])
              n229 = Logarithm Base 10(1:w436) -> (0:w437:dbl[])
            }
          }
          n230 = Bundle(w430, w426) -> (w432:cluster{dbl[], dbl[]})  [unwired: 1 in]
        }
        "XY Graph" <- w424
        n231 = Index Array(array=w422, index=0) -> (element=w420:i32)
        n232 = property on="XY Graph" class="XYGraph (strict)"("LegNumRows"=w420) -> ()  [unwired: 2 in, 2 out]
      }
      frame #1 {
        n233 = for {
          tunnel: w472 -> [w473] mode=indexing
          i -> [w474]
          n234 = property on="XY Graph" class="XYGraph (strict)"("Active Plot"=w474, "Plot.Plot Name"=w473) -> ()  [unwired: 2 in, 2 out]
        }
      }
    }
    "Global Stop" <- "Finish"
  }
  n235 = Strip Path(path="Fequency sweep datafile") -> (stripped path=w6:path, name=w10:string)
  n236 = Concatenate Strings(w10, "_1.dat") -> (w7:string)
  n237 = while {
    shift-right: [w478] -> _
    shift-left: w7 -> [w488]
    tunnel: w6 -> [w477]
    stop <- "Stop" continue-if-true
    (unwired) FALSE ("Save current freq scan")
    w490 = dbl[] []
    w493 = dbl[] []
    n238 = Tick Count (ms)() -> (millisecond timer value=w492:u32)
    n239 = while {
      shift-right: [w514] -> w475
      shift-left: w493 -> [w512]
      shift-right: [w515] -> w476
      shift-left: w493 -> [w511]
      shift-right: [w536] -> _
      shift-left: _ -> [w537]
      tunnel: [w539] -> _
      tunnel: w492 -> [w531]
      shift-right: [w510] -> _
      shift-left: 0 -> [w529]
      shift-right: [w519] -> _
      shift-left: w490 -> [w518]
      shift-right: [w517] -> _
      shift-left: w490 -> [w520]
      i -> [w516]
      stop <- w513 continue-if-true
      n240 = global read "MQM Data Transfer_KM.vi" "ZI HFLI"() -> (w542:T5)
      n241 = Wait (ms)(milliseconds to wait="DAQ time (ms)") -> ()  [unwired: 1 out]
      n242 = Tick Count (ms)() -> (millisecond timer value=w533:u32)
      n243 = Unbundle By Name(w542) -> ("Lockin 1 Demod 0.Frequency (Hz)"=w536:dbl, "Lockin 1 Demod 0.Theta (deg)"=w538:dbl)
      n244 = Subtract(x=w533, y=w531) -> (x-y=w510:u32)
      n245 = global read "MQM Data Transfer_KM.vi" "ZI HFLI"() -> (w524:T5)
      n246 = Subtract(x=w510, y=w529) -> (x-y=→"Data Rate  (ms)":u32)
      n247 = Unbundle By Name(w524) -> ("Lockin 1 Demod 0.X (mV)"=w522:dbl, "Lockin 1 Demod 0.Y (mV)"=w521:dbl)
      n248 = Add(x=w536, y=1) -> (x+y=w535:dbl)
      n249 = Build Array (concatenate)(w511, w536) -> (w544:dbl[])
      n250 = Greater?(x=w535, y=w537) -> (0:w513:bool)
      n251 = Build Array (concatenate)(w512, w538) -> (w543:dbl[])
      n252 = case shown="2" "Frequency" {
        tunnel: w544 -> [w565 w567 w570]
        tunnel: [w565 w566 w569] -> w515
        frame 0, Default {
        }
        frame 1 {
          n253 = Reciprocal(x=w567) -> (1/x=w566:dbl[])
        }
        frame 2 {
          n254 = Absolute Value(x=w570) -> (abs(x)=w568:dbl[])
          n255 = Logarithm Base 10(1:w568) -> (0:w569:dbl[])
        }
      }
      n256 = case shown="0, Default" "Theta" {
        tunnel: [w559 w561 w564] -> w514
        tunnel: w543 -> [w559 w560 w562]
        frame 0, Default {
        }
        frame 1 {
          n257 = Reciprocal(x=w560) -> (1/x=w561:dbl[])
        }
        frame 2 {
          n258 = Absolute Value(x=w562) -> (abs(x)=w563:dbl[])
          n259 = Logarithm Base 10(1:w563) -> (0:w564:dbl[])
        }
      }
      n260 = Build Array (concatenate)(w518, w522) -> (w526:dbl[])
      n261 = Build Array (concatenate)(w520, w521) -> (w525:dbl[])
      n262 = case shown="2" "X" {
        tunnel: w526 -> [w553 w555 w558]
        tunnel: [w553 w554 w557] -> w519
        frame 0, Default {
        }
        frame 1 {
          n263 = Reciprocal(x=w555) -> (1/x=w554:dbl[])
        }
        frame 2 {
          n264 = Absolute Value(x=w558) -> (abs(x)=w556:dbl[])
          n265 = Logarithm Base 10(1:w556) -> (0:w557:dbl[])
        }
      }
      n266 = case shown="0, Default" "Y" {
        tunnel: [w547 w549 w552] -> w517
        tunnel: w525 -> [w547 w548 w550]
        frame 0, Default {
        }
        frame 1 {
          n267 = Reciprocal(x=w548) -> (1/x=w549:dbl[])
        }
        frame 2 {
          n268 = Absolute Value(x=w550) -> (abs(x)=w551:dbl[])
          n269 = Logarithm Base 10(1:w551) -> (0:w552:dbl[])
        }
      }
      n270 = Divide(x=w515, y=1000) -> (x/y=w540:dbl[])
      n271 = Bundle(w540, w514) -> (w539:cluster{dbl[], dbl[]})  [unwired: 1 in]
      "Phase" <- w539
      n272 = Bundle(w519, w517) -> (→"Circles":cluster{dbl[], dbl[]})  [unwired: 1 in]
      "# pts in freq sweep" <- w516
    }
    n273 = local write "Save current freq scan"(FALSE) -> ()
    n274 = case shown="True" "Save current freq scan" {
      tunnel: [w495 w497] -> w478
      tunnel: w488 -> [w495 w496]
      frame False {
      }
      frame True {
        n275 = Search/Split String(string=w496, search string/char (-)="_") -> (substring before match=w508:string, match + rest of string=w507:string)  [unwired: 1 in, 1 out]
        n276 = Decimal String To Number(string=w507, offset=1) -> (number=w505:i32)  [unwired: 1 in, 1 out]
        n277 = Add(x=w505, y=1) -> (x+y=w502:i32)
        n278 = Number To Fractional String(use system decimal point (T)=FALSE, number=w502, precision (6)=0) -> (F-format string=w501:string)  [unwired: 1 in]
        n279 = Concatenate Strings(w508, "_", w501, ".dat") -> (w497:string)
      }
    }
    n280 = Build Path(base path=w477, name or relative path=w478) -> (appended path=w486:path)
    n281 = Build Array(w476, w475) -> (w484:dbl[][])
    n282 = Transpose 2D Array(2D array=w484) -> (transposed array=w485:dbl[][])
    n283 = call-poly <vilib>:"Write To Spreadsheet File.vi"("append to file? (new file:F)"=FALSE, "1D data"=string[] ["Frequency (Hz) ", "Theta (deg)"], "file path (dialog if empty)"=w486) -> ("new file path (Not A Path if cancelled)"=w480:path)  [unwired: 5 in]
    n284 = call-poly <vilib>:"Write To Spreadsheet File.vi"("format (%.3f)"="%.8f", "append to file? (new file:F)"=TRUE, "2D data"=w485, "file path (dialog if empty)"=w480) -> ()  [unwired: 4 in, 1 out]
  }
  n285 = call "ControlHFLI.vi"("Sweep"="Control", "Bandwidth (Hz)"="Bandwidth (Hz)", "Number of Points"="# pts in scan", "Stop (Hz)"="Stop (Hz)", "Start (Hz)"="Start (Hz)") -> ()  [unwired: 7 in]
